vi "cource ns us ns LV.vi"(0 "sec in":i32, 5 "ms in":i32, 7 "µs in":i32, 9 "ns in":i32, 11 "ps in":i32 min=-1000 max=1000) -> (4 "sec out":i32, 6 "ms out":i32, 8 "µs out":i32, 10 "ns out":i32, 15 "ps out":i32)   [LabVIEW 2009, in "CS POLARIS BME DG Client.lvlib"]
uses:
  CS POLARIS BME DG Client.lvlib
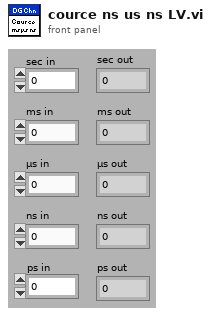
[diagram p1: front panel]
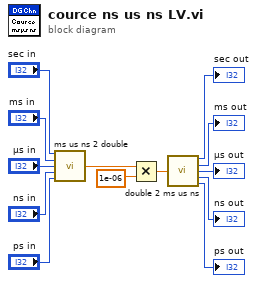
[diagram p0: block diagram]
diagram:
  n1 = call "ms us ns 2 double.vi"("sec"="sec in", "ms"="ms in", "µs"="µs in", "ns"="ns in", "ps"="ps in") -> ("µs"=w10:dbl)  [unwired: 10 in]
  n2 = Multiply(x=w10, y=1e-06) -> (x*y=w12:dbl)
  n3 = call "double 2 ms us ns.vi"("sec"=w12) -> ("sec"=→"sec out":i32, "ms"=→"ms out":i32, "µs"=→"µs out":i32, "ns"=→"ns out":i32, "ps"=→"ps out":i32)  [unwired: 10 in]
